vi "写入excel(幅值线性度).vi"(7 "设置":string[](array[string])=["160", "10", "0.02", "0.02", "0.1", "10", "J5", "J6"], 8 "error in (no error)":errorcluster, 9 "被测幅值":dbl[](array[numeric]), 10 "参考幅值":dbl format="%.2p", 11 "NI_report输入":refnum<class "NI_report.lvclass">) -> (0 "error out":errorcluster, 3 "report out":refnum<class "NI_report.lvclass">)   [LabVIEW 2015]
uses:
  <vilib>/Utility/NIReport.llb/NI_report.lvclass
  <vilib>/addons/_office/_exclsub.llb/font.ctl
  Global.vi
  <vilib>/Utility/NIReport.llb/Excel/NI_Excel.lvclass
  <vilib>/addons/_office/NI_ReportGenerationToolkit.lvlib
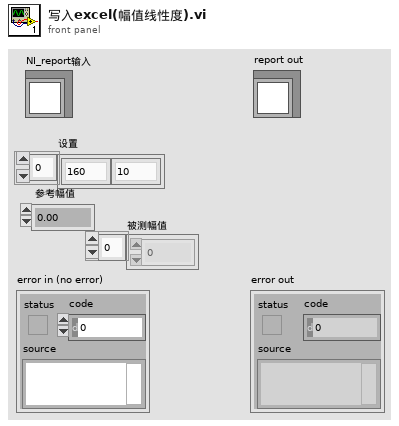
[diagram p1: front panel]
types:
  T1 = typedef "NI_ReportGenerationToolkit.lvlib/font.ctl" = cluster{"font name":string, "font size":dbl, "bold":u16, "italic":u16, "underline":u16, "strike through":u16, "font color":u32}
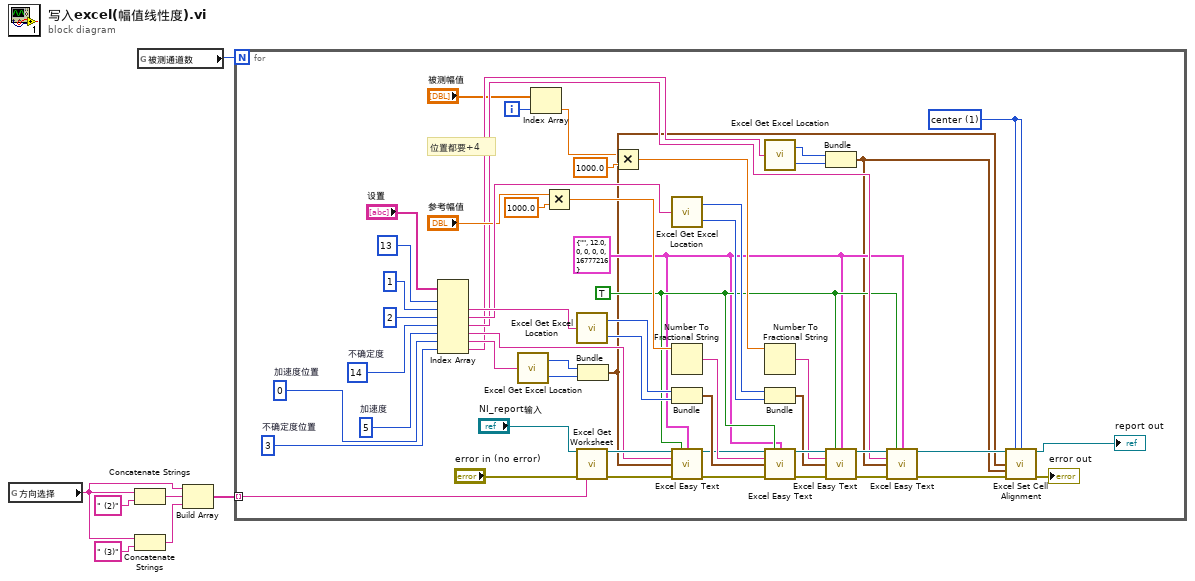
[diagram p0: block diagram]
diagram:
  n1 = global read "Global.vi" "方向选择"() -> (w4:string)
  n2 = Concatenate Strings(w4, " (2)") -> (w5:string)
  n3 = Concatenate Strings(w4, " (3)") -> (w6:string)
  n4 = global read "Global.vi" "被测通道数"() -> (w7:i32)
  n5 = Build Array(w4, w5, w6) -> (w1:string[])
  n6 = for {
    N: w7 -> [_]
    tunnel: w1 -> [w8] mode=indexing
    i -> [w10]
    w19 = 3  # 不确定度位置
    w33 = 0  # 加速度位置
    w34 = 5  # 加速度
    w35 = 14  # 不确定度
    w41 = 1 items=["top", "center", "bottom"] ("vertical alignment (top)")
    w15 = TRUE ("border? (F)")
    w14 = T1 {"font name"="", "font size"=12.0, "bold"=0, "italic"=0, "underline"=0, "strike through"=0, "font color"=16777216} ("font")
    # "位置都要+4"
    n7 = Index Array(array="设置", index #1=13 ("索引"), index #2=1 ("索引 (行)"), index #3=2 ("索引"), index #4=w35, index #5=w34, index #6=w33, index #7=w19) -> (element #2=w54:string, element #3=w48:string, element #4=w20:string, element #5=w30:string, element #6=w29:string, element #7=w18:string)  [unwired: 1 out]
    n8 = call <vilib>:"Excel Get Excel Location.vi"("cell's name"=w29) -> ("row"=w28:i32, "column"=w27:i32)
    n9 = Index Array(array="被测幅值", index=w10) -> (element=w9:dbl)
    n10 = Multiply(x="参考幅值", y=1000.0) -> (x*y=w36:dbl)
    n11 = call <vilib>:"Excel Get Excel Location.vi"("cell's name"=w54) -> ("row"=w53:i32, "column"=w52:i32)
    n12 = call <vilib>:"Excel Get Worksheet.vi"("report in"="NI_report输入", "error in (no error)"="error in (no error)", "name (\"\")"=w8) -> ("report out"=w32:refnum<class "NI_report.lvclass">, "error out"=w31:errorcluster)  [unwired: 11 in]
    n13 = Bundle("row"=w28, "column"=w27) -> (w13:cluster{"row":i32, "column":i32})  [unwired: 1 in]
    n14 = Multiply(x=w9, y=1000.0) -> (x*y=w39:dbl)
    n15 = call <vilib>:"Excel Get Excel Location.vi"("cell's name"=w48) -> ("row"=w47:i32, "column"=w46:i32)
    n16 = Number To Fractional String(number=w36) -> (F-format string=w55:string)  [unwired: 3 in]
    n17 = Bundle("row"=w53, "column"=w52) -> (w43:cluster{"row":i32, "column":i32})  [unwired: 1 in]
    n18 = call <vilib>:"Excel Easy Text.vi"("report in"=w32, "border? (F)"=w15, "font"=w14, "text"=w30, "start (-1, -1)"=w13, "error in (no error)"=w31) -> ("report out"=w26:refnum<class "NI_report.lvclass">, "error out"=w25:errorcluster)  [unwired: 5 in, 3 out]
    n19 = call <vilib>:"Excel Get Excel Location.vi"("cell's name"=w18) -> ("row"=w17:i32, "column"=w16:i32)
    n20 = Number To Fractional String(number=w39) -> (F-format string=w49:string)  [unwired: 3 in]
    n21 = Bundle("row"=w47, "column"=w46) -> (w42:cluster{"row":i32, "column":i32})  [unwired: 1 in]
    n22 = call <vilib>:"Excel Easy Text.vi"("report in"=w26, "border? (F)"=w15, "font"=w14, "text"=w55, "start (-1, -1)"=w43, "error in (no error)"=w25) -> ("report out"=w51:refnum<class "NI_report.lvclass">, "error out"=w50:errorcluster)  [unwired: 5 in, 3 out]
    n23 = Bundle("row"=w17, "column"=w16) -> (w12:cluster{"row":i32, "column":i32})  [unwired: 1 in]
    n24 = call <vilib>:"Excel Easy Text.vi"("report in"=w51, "border? (F)"=w15, "font"=w14, "text"=w49, "start (-1, -1)"=w42, "error in (no error)"=w50) -> ("report out"=w24:refnum<class "NI_report.lvclass">, "error out"=w23:errorcluster)  [unwired: 5 in, 3 out]
    n25 = call <vilib>:"Excel Easy Text.vi"("report in"=w24, "border? (F)"=w15, "font"=w14, "text"=w20, "start (-1, -1)"=w12, "error in (no error)"=w23) -> ("report out"=w22:refnum<class "NI_report.lvclass">, "error out"=w21:errorcluster)  [unwired: 5 in, 3 out]
    n26 = call <vilib>:"Excel Set Cell Alignment.vi"("report in"=w22, "vertical alignment (top)"=w41, "horizontal alignment (left)"=w41, "start (-1, -1)"=w13, "end (-1, -1)"=w12, "error in (no error)"=w21) -> ("report out"=→"report out":refnum<class "NI_report.lvclass">, "error out"=→"error out":errorcluster)  [unwired: 8 in]
  }
